vi "SaveBGorCali(SubVI).vi"(0 "Channel1":cluster{"2DRawDataIn":dbl[][], "CtrlV":dbl[]}, 1 "BG path":path, 3 "DataType":enum16{"BG", "Cali"}(ring), 5 "Channel 2":cluster{"2DRawDataIn":dbl[][], "CtrlV":dbl[]}, 7 "Channel 3":cluster{"2DRawDataIn":dbl[][], "CtrlV":dbl[]}, 9 "Channel 4":cluster{"2DRawDataIn":dbl[][], "CtrlV":dbl[]}, 11 "error in (no error)":errorcluster, 12 "SytemID":string(combo)="UCDMC") -> (15 "error out":errorcluster)   [LabVIEW 2024]
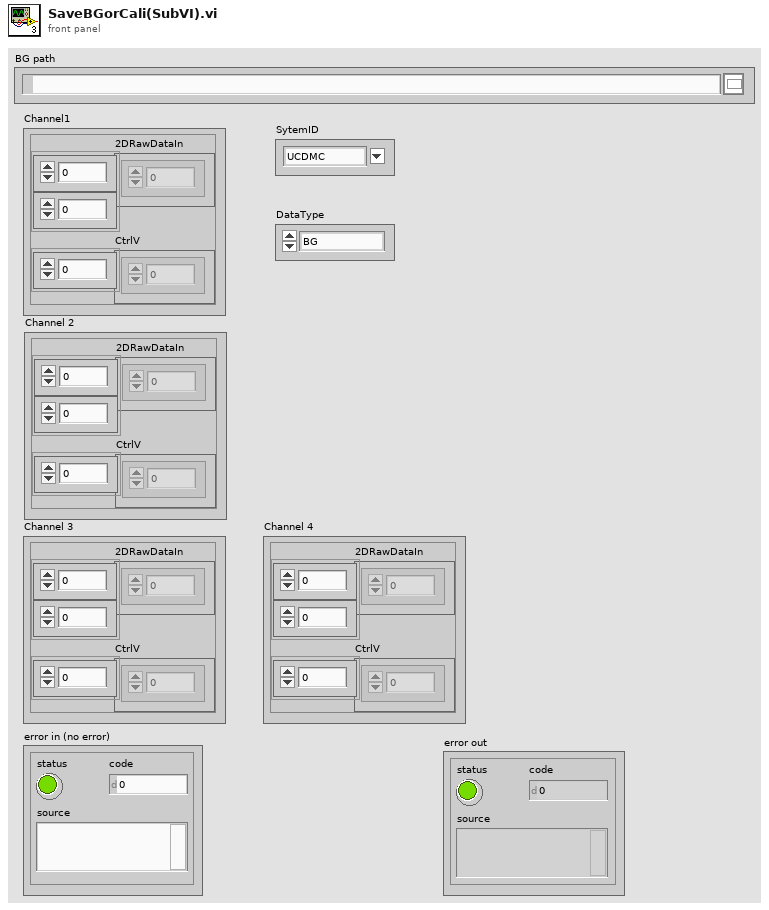
[diagram p1: front panel]
types:
  T1 = enum16{"open", "open or create", "create or replace", "create", "open (read-only)"}
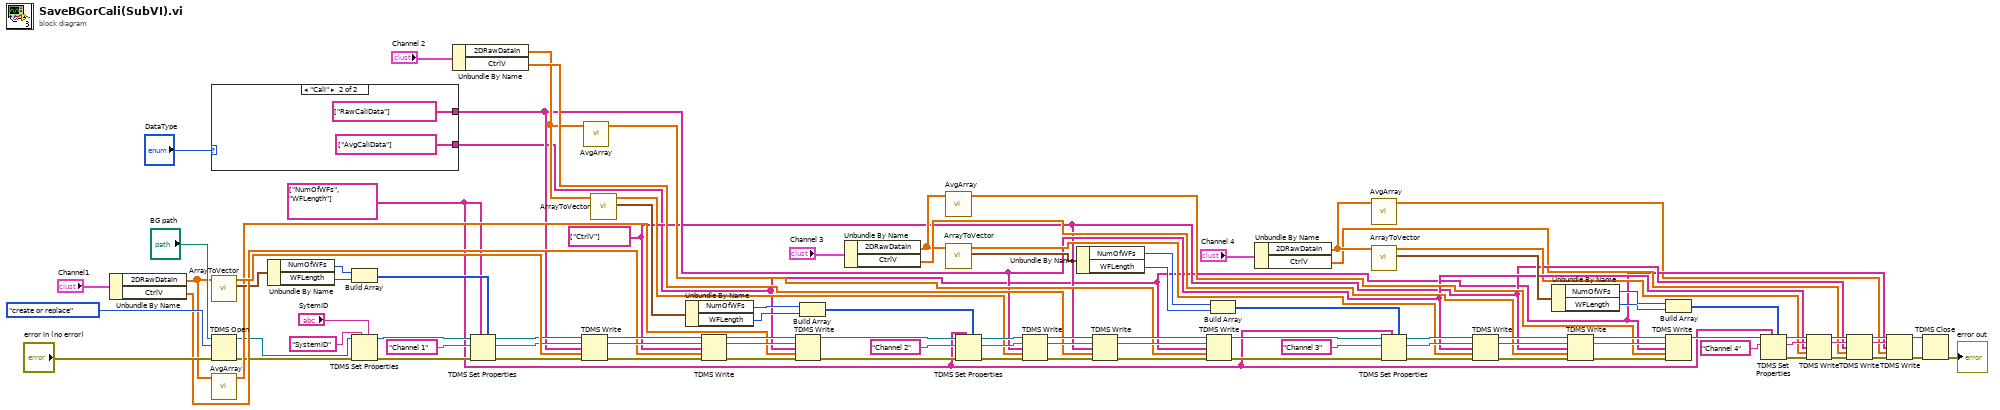
[diagram p0: block diagram]
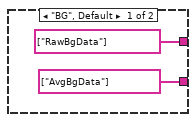
[diagram p2: hidden frame]
diagram:
  w6 = string[] ["CtrlV"] ("channel name(s) in (Untitled)")
  w11 = string[] ["NumOfWFs", "WFLength"] ("property names")
  n1 = Unbundle By Name("Channel1") -> ("2DRawDataIn"=w52:dbl[][], "CtrlV"=w87:dbl[])
  n2 = case shown="\"Cali\"" "DataType" {
    tunnel: [string[] ["RawBgData"] ("channel name(s) in (Untitled)") string[] ["RawCaliData"] ("channel name(s) in (Untitled)")] -> w8
    tunnel: [string[] ["AvgBgData"] ("channel name(s) in (Untitled)") string[] ["AvgCaliData"] ("channel name(s) in (Untitled)")] -> w4
    frame "BG", Default {
    }
    frame "Cali" {
    }
  }
  n3 = call "ArrayToVector.vi"("2D WF in"=w52) -> ("WF Dimension"=w66:cluster{"NumOfWFs":i32, "WFLength":i32}, "1D WF out"=w93:dbl[])  [unwired: 9 in]
  n4 = TDMS Open(8:"error in (no error)", 10:T1."create or replace" ("operation (0:open)"), 11:"BG path") -> (0:w32:errorcluster, 3:w33:refnum<k34>)  [unwired: 4 in]
  n5 = call "AvgArray.vi"("2D array in"=w52) -> ("1D Avg out"=w48:dbl[])  [unwired: 10 in]
  n6 = Unbundle By Name(w66) -> ("NumOfWFs"=w65:i32, "WFLength"=w64:i32)
  n7 = Build Array(w65, w64) -> (w63:i32[])
  n8 = TDMS Set Properties(5:"SytemID", 7:"SystemID" ("group name in (Untitled)"), 8:w32, 11:w33) -> (0:w30:errorcluster, 3:w31:refnum<k34>)  [unwired: 2 in, 2 out]
  n9 = Unbundle By Name("Channel 2") -> ("2DRawDataIn"=w40:dbl[][], "CtrlV"=w76:dbl[])
  n10 = TDMS Set Properties(5:w63, 7:w11, 8:w30, 10:"Channel 1" ("group name in (Untitled)"), 11:w31) -> (0:w91:errorcluster, 2:w82:string, 3:w92:refnum<k34>)  [unwired: 1 in, 1 out]
  n11 = TDMS Write(0:w92, 5:w82, 7:w8, 9:w93, 11:w91) -> (4:w89:refnum<k34>, 6:w90:string, 15:w88:errorcluster)  [unwired: 1 in, 1 out]
  n12 = call "AvgArray.vi"("2D array in"=w40) -> ("1D Avg out"=w39:dbl[])  [unwired: 10 in]
  n13 = call "ArrayToVector.vi"("2D WF in"=w40) -> ("WF Dimension"=w61:cluster{"NumOfWFs":i32, "WFLength":i32}, "1D WF out"=w62:dbl[])  [unwired: 9 in]
  n14 = Unbundle By Name(w61) -> ("NumOfWFs"=w60:i32, "WFLength"=w59:i32)
  n15 = TDMS Write(0:w89, 5:w90, 7:w6, 9:w87, 11:w88) -> (4:w51:refnum<k34>, 6:w49:string, 15:w50:errorcluster)  [unwired: 1 in, 1 out]
  n16 = TDMS Write(0:w51, 5:w49, 7:w4, 9:w48, 11:w50) -> (4:w47:refnum<k34>, 15:w46:errorcluster)  [unwired: 1 in, 2 out]
  n17 = Build Array(w60, w59) -> (w58:i32[])
  n18 = Unbundle By Name("Channel 3") -> ("2DRawDataIn"=w38:dbl[][], "CtrlV"=w67:dbl[])
  n19 = call "AvgArray.vi"("2D array in"=w38) -> ("1D Avg out"=w35:dbl[])  [unwired: 10 in]
  n20 = call "ArrayToVector.vi"("2D WF in"=w38) -> ("WF Dimension"=w56:cluster{"NumOfWFs":i32, "WFLength":i32}, "1D WF out"=w57:dbl[])  [unwired: 9 in]
  n21 = TDMS Set Properties(5:w58, 7:w11, 8:w46, 10:"Channel 2" ("group name in (Untitled)"), 11:w47) -> (0:w80:errorcluster, 2:w81:string, 3:w84:refnum<k34>)  [unwired: 1 in, 1 out]
  n22 = TDMS Write(0:w84, 5:w81, 7:w8, 9:w62, 11:w80) -> (4:w79:refnum<k34>, 6:w77:string, 15:w78:errorcluster)  [unwired: 1 in, 1 out]
  n23 = Unbundle By Name(w56) -> ("NumOfWFs"=w55:i32, "WFLength"=w54:i32)
  n24 = TDMS Write(0:w79, 5:w77, 7:w6, 9:w76, 11:w78) -> (4:w45:refnum<k34>, 6:w44:string, 15:w43:errorcluster)  [unwired: 1 in, 1 out]
  n25 = TDMS Write(0:w45, 5:w44, 7:w4, 9:w39, 11:w43) -> (4:w42:refnum<k34>, 15:w41:errorcluster)  [unwired: 1 in, 2 out]
  n26 = Build Array(w55, w54) -> (w53:i32[])
  n27 = Unbundle By Name("Channel 4") -> ("2DRawDataIn"=w25:dbl[][], "CtrlV"=w5:dbl[])
  n28 = call "AvgArray.vi"("2D array in"=w25) -> ("1D Avg out"=w3:dbl[])  [unwired: 10 in]
  n29 = call "ArrayToVector.vi"("2D WF in"=w25) -> ("WF Dimension"=w24:cluster{"NumOfWFs":i32, "WFLength":i32}, "1D WF out"=w7:dbl[])  [unwired: 9 in]
  n30 = TDMS Set Properties(5:w53, 7:w11, 8:w41, 10:"Channel 3" ("group name in (Untitled)"), 11:w42) -> (0:w73:errorcluster, 2:w69:string, 3:w74:refnum<k34>)  [unwired: 1 in, 1 out]
  n31 = TDMS Write(0:w74, 5:w69, 7:w8, 9:w57, 11:w73) -> (4:w72:refnum<k34>, 6:w68:string, 15:w71:errorcluster)  [unwired: 1 in, 1 out]
  n32 = Unbundle By Name(w24) -> ("NumOfWFs"=w23:i32, "WFLength"=w22:i32)
  n33 = TDMS Write(0:w72, 5:w68, 7:w6, 9:w67, 11:w71) -> (4:w37:refnum<k34>, 6:w36:string, 15:w34:errorcluster)  [unwired: 1 in, 1 out]
  n34 = Build Array(w23, w22) -> (w10:i32[])
  n35 = TDMS Write(0:w37, 5:w36, 7:w4, 9:w35, 11:w34) -> (4:w12:refnum<k34>)  [unwired: 1 in, 3 out]
  n36 = TDMS Set Properties(5:w10, 7:w11, 10:"Channel 4" ("group name in (Untitled)"), 11:w12) -> (0:w20:errorcluster, 2:w17:string, 3:w21:refnum<k34>)  [unwired: 2 in, 1 out]
  n37 = TDMS Write(0:w21, 5:w17, 7:w8, 9:w7, 11:w20) -> (4:w19:refnum<k34>, 6:w16:string, 15:w18:errorcluster)  [unwired: 1 in, 1 out]
  n38 = TDMS Write(0:w19, 5:w16, 7:w6, 9:w5, 11:w18) -> (4:w15:refnum<k34>, 6:w14:string, 15:w13:errorcluster)  [unwired: 1 in, 1 out]
  n39 = TDMS Write(0:w15, 5:w14, 7:w4, 9:w3, 11:w13) -> (4:w1:refnum<k34>, 15:w2:errorcluster)  [unwired: 1 in, 2 out]
  n40 = TDMS Close(8:w2, 11:w1) -> (0:→"error out":errorcluster)  [unwired: 1 out]
